vi "kiethleyRef.vi"() -> ()   [LabVIEW 2019]
panel:
  in  "VISA resource name":refnum<visa-resource-name>
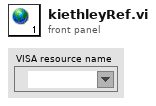
[diagram p1: front panel]
diagram:
